vi "rename custom device xml.vi"(8 "error in":errorcluster, 10 "User Project":refnum<vi>, 11 "CD name":string) -> (0 "error out":errorcluster, 3 "new xml path":path)   [LabVIEW 2014, in "CD model script.lvlib"]
uses:
  CD model script.lvlib
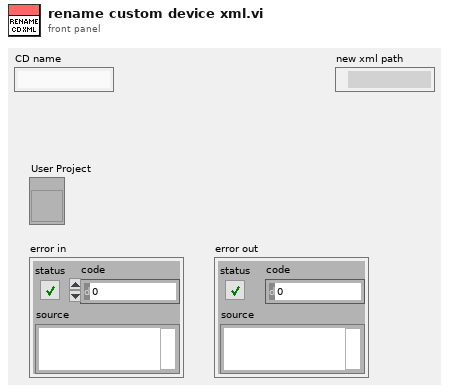
[diagram p1: front panel]
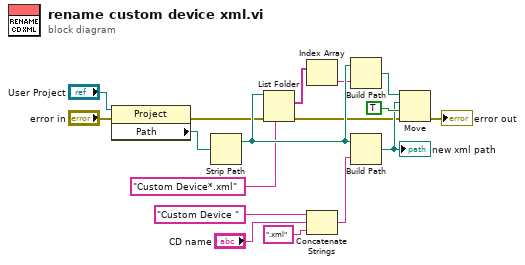
[diagram p0: block diagram]
diagram:
  n1 = property class="Project"(reference="User Project", error in="error in") -> (error out=w3:errorcluster, "Path"=w5:path)  [unwired: 1 out]
  n2 = Strip Path(path=w5) -> (stripped path=w12:path)  [unwired: 1 out]
  n3 = List Folder(path=w12, pattern="Custom Device*.xml", error in=w3) -> (filenames=w8:string[], error out=w6:errorcluster)  [unwired: 1 in, 2 out]
  n4 = Index Array(array=w8) -> (element=w11:string)  [unwired: 1 in]
  n5 = Concatenate Strings("Custom Device " ("string"), "CD name", ".xml" ("string")) -> (w13:string)
  n6 = Build Path(base path=w12, name or relative path=w11) -> (appended path=w15:path)
  n7 = Build Path(base path=w12, name or relative path=w13) -> (appended path=w16:path)
  "new xml path" <- w16
  n8 = Move(source path=w15, error in=w6, 9:TRUE ("overwrite (F)"), 10:w16) -> (error out=→"error out":errorcluster)  [unwired: 1 in, 2 out]
